vi "Vision_ExecLogic.vi"() -> ()   [LabVIEW 2025]
uses:
  <vilib>/Rock Robotics/WPI/ThirdParty/PhotonVisionLib/Enum/PhotonPoseStrategy_ENUM.ctl
  <vilib>/Rock Robotics/WPI/ThirdParty/JAS_Junk/TrajLib/VI/AprilTagFieldLayout_New2026Welded.vi
  <vilib>/Rock Robotics/WPI/ThirdParty/PhotonVisionLib/SubVI/PhotonPipelineResult_Unpack.vi
  <vilib>/Rock Robotics/WPI/ThirdParty/PhotonVisionLib/SubVI/PhotonPipelineResult_GetMetadata.vi
  <vilib>/Rock Robotics/WPI/ThirdParty/PhotonVisionLib/SubVI/PhotonPipelineMetadata_GetAll.vi
  <vilib>/Rock Robotics/WPI/ThirdParty/PhotonVisionLib/SubVI/PhotonPipelineResult_HasTargets.vi
  <vilib>/Rock Robotics/WPI/ThirdParty/JAS_Junk/TrajLib/VI/Quaternion_New.vi
  <vilib>/Rock Robotics/WPI/ThirdParty/JAS_Junk/TrajLib/VI/AprilTagFieldLayout_New.vi
  <vilib>/Rock Robotics/WPI/ThirdParty/JAS_Junk/TrajLib/VI/Pose3d_New_Trans3dRot3d.vi
  <vilib>/Rock Robotics/WPI/ThirdParty/JAS_Junk/TrajLib/VI/Rotation3d_Create_Quaternion.vi
  <vilib>/Rock Robotics/WPI/ThirdParty/JAS_Junk/TrajLib/VI/AprilTag_New.vi
  <vilib>/Rock Robotics/WPI/ThirdParty/JAS_Junk/TrajLib/VI/Transform3d_Equals.vi
  <vilib>/Rock Robotics/WPI/ThirdParty/PhotonVisionLib/SubVI/PhotonPoseEstimator_SetCamera.vi
  <vilib>/Rock Robotics/WPI/ThirdParty/PhotonVisionLib/SubVI/PhotonPoseEstimator_SetPrimaryStategy.vi
  <vilib>/Rock Robotics/WPI/ThirdParty/PhotonVisionLib/SubVI/PhotonPoseEstimator_SetMultiTagFallbackStrategy.vi
  <vilib>/Rock Robotics/WPI/ThirdParty/PhotonVisionLib/SubVI/PhotonPoseEstimator_SetHighestAmbiguity.vi
  <vilib>/Rock Robotics/WPI/ThirdParty/PhotonVisionLib/SubVI/PhotonPoseEstimator_SetRobotToCameraTransform.vi
  <vilib>/Rock Robotics/WPI/ThirdParty/PhotonVisionLib/SubVI/PhotonPoseEstimator_New.vi
  <vilib>/Rock Robotics/WPI/ThirdParty/PhotonVisionLib/SubVI/PhotonPoseEstimator_SetLastPose.vi
  <vilib>/Rock Robotics/WPI/ThirdParty/PhotonVisionLib/SubVI/PhotonPoseEstimator_SetReferencePose.vi
  <vilib>/Rock Robotics/WPI/ThirdParty/PhotonVisionLib/SubVI/PhotonPoseEstimator_Update_MultiTagOnCoproc.vi
  <vilib>/Rock Robotics/WPI/ThirdParty/PhotonVisionLib/SubVI/PhotonEstimatedRobotPose_GetAll.vi
  <vilib>/Rock Robotics/WPI/ThirdParty/JAS_Junk/TrajLib/VI/Pose3d_ToPose2d.vi
  <vilib>/Rock Robotics/WPI/ThirdParty/PhotonVisionLib/SubVI/Packet_decode_ByteI8.vi
  <vilib>/Rock Robotics/WPI/ThirdParty/PhotonVisionLib/SubVI/PhotonTrackedTarget_Unpack.vi
  <vilib>/Rock Robotics/WPI/ThirdParty/PhotonVisionLib/SubVI/PhotonMultiTargetPNPResult_unpack.vi
  <vilib>/Rock Robotics/WPI/ThirdParty/PhotonVisionLib/SubVI/PhotonPipelineMetadata_Unpack.vi
  <vilib>/Rock Robotics/WPI/ThirdParty/PhotonVisionLib/SubVI/PhotonPipelineResult_New.vi
  <vilib>/Rock Robotics/WPI/ThirdParty/PhotonVisionLib/SubVI/PhotonPipelineResult_GetTargetCount.vi
  <vilib>/Rock Robotics/WPI/ThirdParty/JAS_Junk/TrajLib/VI/AprilTag_GetAll.vi
  <vilib>/Rock Robotics/WPI/ThirdParty/JAS_Junk/TrajLib/VI/Quaternion_Normalize.vi
  <vilib>/Rock Robotics/WPI/ThirdParty/JAS_Junk/TrajLib/VI/Transform3d_GetTranslation3d.vi
  <vilib>/Rock Robotics/WPI/ThirdParty/JAS_Junk/TrajLib/VI/Transform3d_GetRotation3d.vi
  <vilib>/Rock Robotics/WPI/ThirdParty/JAS_Junk/TrajLib/VI/Rotation3d_Equals.vi
  <vilib>/Rock Robotics/WPI/ThirdParty/JAS_Junk/TrajLib/VI/Translation3d_Equals.vi
  <vilib>/Rock Robotics/WPI/ThirdParty/PhotonVisionLib/SubVI/PhotonTargetModel_New_AprilTag36H11.vi
  <vilib>/Rock Robotics/WPI/ThirdParty/JAS_Junk/TrajLib/VI/TimeInterpRotation2d_New.vi
  <vilib>/Rock Robotics/WPI/ThirdParty/PhotonVisionLib/SubVI/PhotonPoseEstimator_GetEmptyPose.vi
  <vilib>/Rock Robotics/WPI/ThirdParty/PhotonVisionLib/SubVI/PhotonPoseEstimator_EstimateMultiTagOnCoprocPose.vi
  <vilib>/Rock Robotics/WPI/ThirdParty/PhotonVisionLib/SubVI/PhotonPipelineResult_GetTimeStampSecs.vi
  <vilib>/Rock Robotics/WPI/ThirdParty/PhotonVisionLib/SubVI/PhotonPoseEstimator_EstimateLowestAmbiguityPose.vi
  <vilib>/Rock Robotics/WPI/ThirdParty/PhotonVisionLib/SubVI/PhotonPoseEstimator_EstimateClosestToCameraHeightPose.vi
  <vilib>/Rock Robotics/WPI/ThirdParty/PhotonVisionLib/SubVI/PhotonPoseEstimator_EstimateClosestToReferencePose.vi
  <vilib>/Rock Robotics/WPI/ThirdParty/PhotonVisionLib/SubVI/PhotonPoseEstimator_GetReferencePose.vi
  <vilib>/Rock Robotics/WPI/ThirdParty/PhotonVisionLib/SubVI/PhotonPoseEstimator_GetLastPose.vi
  <vilib>/Rock Robotics/WPI/ThirdParty/PhotonVisionLib/SubVI/PhotonPoseEstimator_EstimateAverageBestTargetsPose.vi
  <vilib>/Rock Robotics/WPI/ThirdParty/PhotonVisionLib/SubVI/PhotonEstimatedRobotPose_New.vi
  <vilib>/Rock Robotics/WPI/ThirdParty/PhotonVisionLib/SubVI/PhotonPoseEstimator_EstimatePnpDistanceTrigSolvePose.vi
  <vilib>/Rock Robotics/WPI/ThirdParty/PhotonVisionLib/SubVI/PhotonPoseEstimator_ShouldEstimate.vi
  <vilib>/Rock Robotics/WPI/ThirdParty/JAS_Junk/TrajLib/VI/Pose3d_getTranslation3d.vi
  <vilib>/Rock Robotics/WPI/ThirdParty/JAS_Junk/TrajLib/VI/Pose3d_getRotation3d.vi
  <vilib>/Rock Robotics/WPI/ThirdParty/JAS_Junk/TrajLib/VI/Translation3d_ToTranslation2d.vi
  <vilib>/Rock Robotics/WPI/ThirdParty/JAS_Junk/TrajLib/VI/Rotation3d_ToRotation2d.vi
  <vilib>/Rock Robotics/WPI/ThirdParty/JAS_Junk/TrajLib/Pose2d_New_TRRO.vi
  <vilib>/Rock Robotics/WPI/ThirdParty/PhotonVisionLib/SubVI/Packet_decode_Flt64.vi
  <vilib>/Rock Robotics/WPI/ThirdParty/PhotonVisionLib/SubVI/TargetCorner_New.vi
  <vilib>/Rock Robotics/WPI/ThirdParty/PhotonVisionLib/SubVI/Packet_decode_Int32.vi
  <vilib>/Rock Robotics/WPI/ThirdParty/PhotonVisionLib/SubVI/Packet_decode_Transform3d.vi
  <vilib>/Rock Robotics/WPI/ThirdParty/PhotonVisionLib/SubVI/Packet_decode_Flt32.vi
  <vilib>/Rock Robotics/WPI/ThirdParty/PhotonVisionLib/SubVI/Packet_decode_TargetCornerArray.vi
  <vilib>/Rock Robotics/WPI/ThirdParty/PhotonVisionLib/SubVI/Packet_decode_Boolean.vi
  <vilib>/Rock Robotics/WPI/ThirdParty/PhotonVisionLib/SubVI/PhotonPNPResult_unpack.vi
  <vilib>/Rock Robotics/WPI/ThirdParty/PhotonVisionLib/SubVI/PhotonMultiTargetPNPResult_New.vi
  <vilib>/Rock Robotics/WPI/ThirdParty/PhotonVisionLib/SubVI/Packet_decode_Int16.vi
  <vilib>/Rock Robotics/WPI/ThirdParty/PhotonVisionLib/SubVI/Packet_decode_Int64.vi
  <vilib>/Rock Robotics/WPI/ThirdParty/JAS_Junk/TrajLib/VI/Quaternion_New_Default.vi
  <vilib>/Rock Robotics/WPI/ThirdParty/JAS_Junk/TrajLib/VI/Rotation3d_GetQuaterion.vi
  <vilib>/Rock Robotics/WPI/ThirdParty/JAS_Junk/TrajLib/VI/Quaternion_Equals.vi
  <vilib>/Rock Robotics/WPI/ThirdParty/PhotonVisionLib/SubVI/PhotonTargetModel_New_RectPlanar.vi
  <vilib>/Rock Robotics/WPI/ThirdParty/JAS_Junk/TrajLib/Conv_Inches_Meters.vi
  <vilib>/Rock Robotics/WPI/ThirdParty/JAS_Junk/TrajLib/VI/Rotation3d_Create_AxisAngle.vi
  <vilib>/Rock Robotics/WPI/ThirdParty/JAS_Junk/TrajLib/VI/Pose3d_New.vi
  <vilib>/Rock Robotics/WPI/ThirdParty/JAS_Junk/TrajLib/VI/Pose3d_New_Default.vi
  <vilib>/Rock Robotics/WPI/ThirdParty/JAS_Junk/TrajLib/VI/Pose3d_Plus.vi
  <vilib>/Rock Robotics/WPI/ThirdParty/JAS_Junk/TrajLib/VI/Pose3d_RelativeTo.vi
  <vilib>/Rock Robotics/WPI/ThirdParty/PhotonVisionLib/SubVI/PhotonPoseEstimator_GetFieldTags.vi
  <vilib>/Rock Robotics/WPI/ThirdParty/JAS_Junk/TrajLib/VI/AprilTagFieldLayout_GetOriginPosition.vi
  <vilib>/Rock Robotics/WPI/ThirdParty/JAS_Junk/TrajLib/VI/Transform3d_Inverse.vi
  <vilib>/Rock Robotics/WPI/ThirdParty/PhotonVisionLib/SubVI/PhotonPoseEstimator_GetRobotToCameraTransform.vi
  <vilib>/Rock Robotics/WPI/ThirdParty/PhotonVisionLib/SubVI/PhotonPipelineResult_GetTargets.vi
  <vilib>/Rock Robotics/WPI/ThirdParty/PhotonVisionLib/SubVI/PhotonPipelineResult_GetMultiTagResult.vi
  <vilib>/Rock Robotics/WPI/ThirdParty/PhotonVisionLib/SubVI/PhotonTrackedTarget_GetPoseAmbiguity.vi
  <vilib>/Rock Robotics/WPI/ThirdParty/PhotonVisionLib/SubVI/PhotonTrackedTarget_GetFiducialId.vi
  <vilib>/Rock Robotics/WPI/ThirdParty/JAS_Junk/TrajLib/VI/AprilTagFieldLayout_GetTagPose.vi
  <vilib>/Rock Robotics/WPI/ThirdParty/JAS_Junk/TrajLib/VI/Pose3d_TransformBy.vi
  <vilib>/Rock Robotics/WPI/ThirdParty/PhotonVisionLib/SubVI/PhotonTrackedTarget_GetBestCameraToTarget.vi
  <vilib>/Rock Robotics/WPI/ThirdParty/PhotonVisionLib/SubVI/PhotonPoseEstimator_GetHighestAmbiguity.vi
  <vilib>/Rock Robotics/WPI/ThirdParty/PhotonVisionLib/SubVI/PhotonPoseEstimator_Strategy_closestToCameraHeight_calc.vi
  <vilib>/Rock Robotics/WPI/ThirdParty/PhotonVisionLib/SubVI/PhotonTrackedTarget_GetAltCameraToTarget.vi
  <vilib>/Rock Robotics/WPI/ThirdParty/PhotonVisionLib/SubVI/PhotonPoseEstimator_Strategy_closestToReferencePose_calc.vi
  <vilib>/Rock Robotics/WPI/ThirdParty/PhotonVisionLib/SubVI/PhotonPoseEstimator_Strategy_averageBestTargets_calc.vi
  <vilib>/Rock Robotics/WPI/ThirdParty/JAS_Junk/TrajLib/VI/Rotation3d_Plus.vi
  <vilib>/Rock Robotics/WPI/ThirdParty/JAS_Junk/TrajLib/VI/Translation3d_Plus.vi
  <vilib>/Rock Robotics/WPI/ThirdParty/JAS_Junk/TrajLib/VI/Translation3d_Times.vi
  <vilib>/Rock Robotics/WPI/ThirdParty/JAS_Junk/TrajLib/VI/Rotation3d_Times.vi
  <vilib>/Rock Robotics/WPI/ThirdParty/JAS_Junk/TrajLib/VI/Rotation3d_Create_Default.vi
  <vilib>/Rock Robotics/WPI/ThirdParty/JAS_Junk/TrajLib/VI/Translation3d_Create_Default.vi
  <vilib>/Rock Robotics/WPI/ThirdParty/JAS_Junk/TrajLib/VI/Translation3d_GetNorm.vi
  <vilib>/Rock Robotics/WPI/ThirdParty/JAS_Junk/TrajLib/VI/Translation3d_Create_DistAng.vi
  <vilib>/Rock Robotics/WPI/ThirdParty/JAS_Junk/TrajLib/VI/Translation3d_RotateBy.vi
  <vilib>/Rock Robotics/WPI/ThirdParty/JAS_Junk/TrajLib/Translation2d_RotateBy.vi
  <vilib>/Rock Robotics/WPI/ThirdParty/JAS_Junk/TrajLib/Pose2d_getTranslation.vi
  <vilib>/Rock Robotics/WPI/ThirdParty/JAS_Junk/TrajLib/Translation2d_Plus.vi
  <vilib>/Rock Robotics/WPI/ThirdParty/JAS_Junk/TrajLib/Translation2d_UnaryMinus.vi
  <vilib>/Rock Robotics/WPI/ThirdParty/JAS_Junk/TrajLib/VI/Pose3d_New_Pose2d.vi
  <vilib>/Rock Robotics/WPI/ThirdParty/JAS_Junk/TrajLib/VI/TimeInterpRotation2d_GetSample.vi
  <vilib>/Rock Robotics/WPI/ThirdParty/PhotonVisionLib/SubVI/PhotonPoseEstimator_GetHeadingBuffer.vi
  <vilib>/Rock Robotics/WPI/ThirdParty/JAS_Junk/TrajLib/Translation2d_Create.vi
  <vilib>/Rock Robotics/WPI/ThirdParty/JAS_Junk/TrajLib/Rotation2d_CreateAngle.vi
  <vilib>/Rock Robotics/WPI/ThirdParty/JAS_Junk/TrajLib/VI/Rotation3d_GetXYZ.vi
  <vilib>/Rock Robotics/WPI/ThirdParty/PhotonVisionLib/SubVI/PhotonPNPResult_New.vi
  <vilib>/Rock Robotics/WPI/ThirdParty/JAS_Junk/TrajLib/VI/Quaternion_Get_Vect.vi
  <vilib>/Rock Robotics/WPI/ThirdParty/JAS_Junk/TrajLib/VI/Quaternion_Get_W.vi
  <vilib>/Rock Robotics/WPI/ThirdParty/PhotonVisionLib/SubVI/PhotonTargetModel_New.vi
  <vilib>/Rock Robotics/WPI/ThirdParty/JAS_Junk/TrajLib/VI/Vector_Norm.vi
  <vilib>/Rock Robotics/WPI/ThirdParty/JAS_Junk/TrajLib/VecBuilder_ArrayBy1Fill.vi
  <vilib>/Rock Robotics/WPI/ThirdParty/JAS_Junk/TrajLib/VI/Transform3d_Create_Pose3dPose3d.vi
  <vilib>/Rock Robotics/WPI/ThirdParty/JAS_Junk/TrajLib/VI/Rotation3d_UnaryMinus.vi
  <vilib>/Rock Robotics/WPI/ThirdParty/JAS_Junk/TrajLib/VI/Translation3d_UnaryMinus.vi
  <vilib>/Rock Robotics/WPI/ThirdParty/JAS_Junk/TrajLib/Transform2d_Create_TransRot.vi
  <vilib>/Rock Robotics/WPI/ThirdParty/JAS_Junk/TrajLib/VI/Transform3d_GetXYZ.vi
  <vilib>/Rock Robotics/WPI/ThirdParty/JAS_Junk/TrajLib/VI/Pose3d_getXYZ.vi
  <vilib>/Rock Robotics/WPI/ThirdParty/PhotonVisionLib/SubVI/PhotonPoseEstimator_CalcDifference.vi
  <vilib>/Rock Robotics/WPI/ThirdParty/JAS_Junk/TrajLib/VI/Rotation3d_RotateBy.vi
  <vilib>/Rock Robotics/WPI/ThirdParty/JAS_Junk/TrajLib/VI/Translation3d_GetXYZ.vi
  <vilib>/Rock Robotics/WPI/ThirdParty/JAS_Junk/TrajLib/VI/Quaternion_Times.vi
  <vilib>/Rock Robotics/WPI/ThirdParty/JAS_Junk/TrajLib/VI/Quaternion_Inverse.vi
  <vilib>/Rock Robotics/WPI/ThirdParty/JAS_Junk/TrajLib/VI/Quaternion_Get_All.vi
  <vilib>/Rock Robotics/WPI/ThirdParty/JAS_Junk/TrajLib/Rotation2d_Interpolate.vi
  <vilib>/Rock Robotics/WPI/ThirdParty/JAS_Junk/TrajLib/MatBuilder_Create.vi
  <vilib>/Rock Robotics/WPI/ThirdParty/JAS_Junk/TrajLib/VI/Translation3d_Minus.vi
  <vilib>/Rock Robotics/WPI/ThirdParty/JAS_Junk/TrajLib/VI/Rotation3d_Minus.vi
  <vilib>/Rock Robotics/WPI/ThirdParty/JAS_Junk/TrajLib/VI/Translation3d_GetDistance.vi
  <vilib>/Rock Robotics/WPI/ThirdParty/JAS_Junk/TrajLib/Rotation2d_Plus.vi
  <vilib>/Rock Robotics/WPI/ThirdParty/JAS_Junk/TrajLib/Rotation2d_Minus.vi
  <vilib>/Rock Robotics/WPI/ThirdParty/JAS_Junk/TrajLib/MathUtil_Clamp.vi
  <vilib>/Rock Robotics/WPI/ThirdParty/JAS_Junk/TrajLib/Rotation2d_Times.vi
  <vilib>/Rock Robotics/WPI/ThirdParty/JAS_Junk/TrajLib/Rotation2d_RotateBy.vi
  <vilib>/Rock Robotics/WPI/ThirdParty/JAS_Junk/TrajLib/Rotation2d_UnaryMinus.vi
  <vilib>/Rock Robotics/WPI/ThirdParty/JAS_Junk/TrajLib/Rotation2d_CreateXY.vi
  <vilib>/Rock Robotics/WPI/ThirdParty/JAS_Junk/TrajLib/Util_CalcDist.vi
  <vilib>/Rock Robotics/Network Tables/NT Read Value.vi
  <vilib>/Rock Robotics/Network Tables/NT Read Raw.vi
  <vilib>/Rock Robotics/WPI/ThirdParty/PhotonVisionLib/SubVI/PhotonVision_Globals.vi
  <vilib>/gmath/interp.llb/Search Ordered Table.vi
  <vilib>/Rock Robotics/Network Tables/NT Write Number.vi
  <vilib>/Rock Robotics/Network Tables/NT Write Boolean.vi
  <vilib>/Rock Robotics/WPI/ThirdParty/PhotonVisionLib/PhotonVisionLib.lvlib
  <vilib>/Rock Robotics/WPI/ThirdParty/JAS_Junk/TrajLib/Trajectory_Library.lvlib
panel:
  in  "Drive Encoder  Dstance (Meters)":dbl
  in  "Gyro Reading (Deg)":dbl
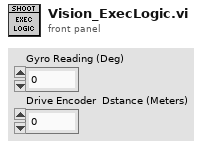
[diagram p1: front panel]
types:
  T1 = typedef "PhotonVisionLib.lvlib/PhotonPoseStrategy_ENUM.ctl" = enum16{"LOWEST_AMBIGUITY", "CLOSEST_TO_CAMERA_HEIGHT", "CLOSEST_TO_REFERENCE_POSE", "CLOSEST_TO_LAST_POSE", "AVERAGE_BEST_TARGETS", "MULTI_TAG_PNP_ON_COPROCESSOR", "MULTI_TAG_PNP_ON_RIO", "PNP_DISTANCE_TRIG_SOLVE", "CONSTRAINED_SOLVEPNP"}
  T2 = typedef "Trajectory_Library.lvlib/TRANSLATION3D.ctl" = cluster{"X":dbl, "Y":dbl, "Z":dbl}
  T3 = typedef "Trajectory_Library.lvlib/AprilTagFieldLayout.ctl" = cluster{"AprilTagMap":map{i32, T4}, "FieldLength":dbl, "FieldWidth":dbl, "OriginPosition ":T8, "OriginPose3d":T5}
  T4 = typedef "Trajectory_Library.lvlib/AprilTag.ctl" = cluster{"ID":i32, "POSE3D":T5}
  T5 = typedef "Trajectory_Library.lvlib/POSE3D.ctl" = cluster{"Translation3d":T2, "Rotation3d":T6}
  T6 = typedef "Trajectory_Library.lvlib/ROTATION3D.ctl" = cluster{"Q_quaternion":T7}
  T7 = typedef "Trajectory_Library.lvlib/QUATERNION.ctl" = cluster{"R":dbl, "V":dbl[]}
  T8 = typedef "Trajectory_Library.lvlib/AprilTagFieldLayoutOrignPosition_ENUM.ctl" = enum16{"kBlueAllianceWallRightSide,", "kRedAllianceWallRightSide,"}
  T9 = typedef "PhotonVisionLib.lvlib/PhotonPipelineResultType.ctl" = cluster{"Targets":T10[], "PhotonMultiTargetPNPResult":T13, "PhotonPipelineMetadata":T15}
  T10 = typedef "PhotonVisionLib.lvlib/PhotonTrackedTargetType.ctl" = cluster{"Yaw":dbl, "Pitch":dbl, "Area":dbl, "Skew":dbl, "MinAreaRectCorners":T11[], "BestCameraToTarget":T12, "FiducialId":i32, "AltCameraToTarget":T12, "PoseAmbiguity":dbl, "DetectedCorners":T11[], "ObjDetectId":i32, "ObjDetectConf":sgl}
  T11 = typedef "PhotonVisionLib.lvlib/TargetCornerType.ctl" = cluster{"X":dbl, "Y":dbl}
  T12 = typedef "Trajectory_Library.lvlib/TRANSFORM3D.ctl" = cluster{"TRANSLATION3D":T2, "ROTATION3D":T6, "XF":bool}
  T13 = typedef "PhotonVisionLib.lvlib/PhotonMultiTargetPNPResultType.ctl" = cluster{"PhotonPNPResult":T14, "FiducialIDsUsed":i16[]}
  T14 = typedef "PhotonVisionLib.lvlib/PhotonPNPResultType.ctl" = cluster{"IsPresent":bool, "bestReprojErr":dbl, "altReprojErr":dbl, "ambiguity":dbl, "Best":T12, "Alt":T12}
  T15 = typedef "PhotonVisionLib.lvlib/PhotonPipelineMetadataType.ctl" = cluster{"CaptureTimestampMicros":i64, "PublishTimestampMicros":i64, "SequenceID":i64, "TimeSinceLastPong":i64}
  T16 = typedef "PhotonVisionLib.lvlib/PhotonPoseEstimator_Configuration.ctl" = cluster{"Primary Strategy":T1, "Camera":string, "Initial Pose":T5, "HighestAmbiguity":dbl, "RobotToCamera":T12, "FallBack Strategy":T1, "BaseNTName":string}
  T17 = typedef "Trajectory_Library.lvlib/POSE2D.ctl" = cluster{"TRANSLATION":T18, "ROTATION":T19}
  T18 = typedef "Trajectory_Library.lvlib/TRANSLATION2D.ctl" = cluster{"X":dbl, "Y":dbl}
  T19 = typedef "Trajectory_Library.lvlib/ROTATION2D.ctl" = cluster{"VALUE":dbl, "COS":dbl, "SIN":dbl}
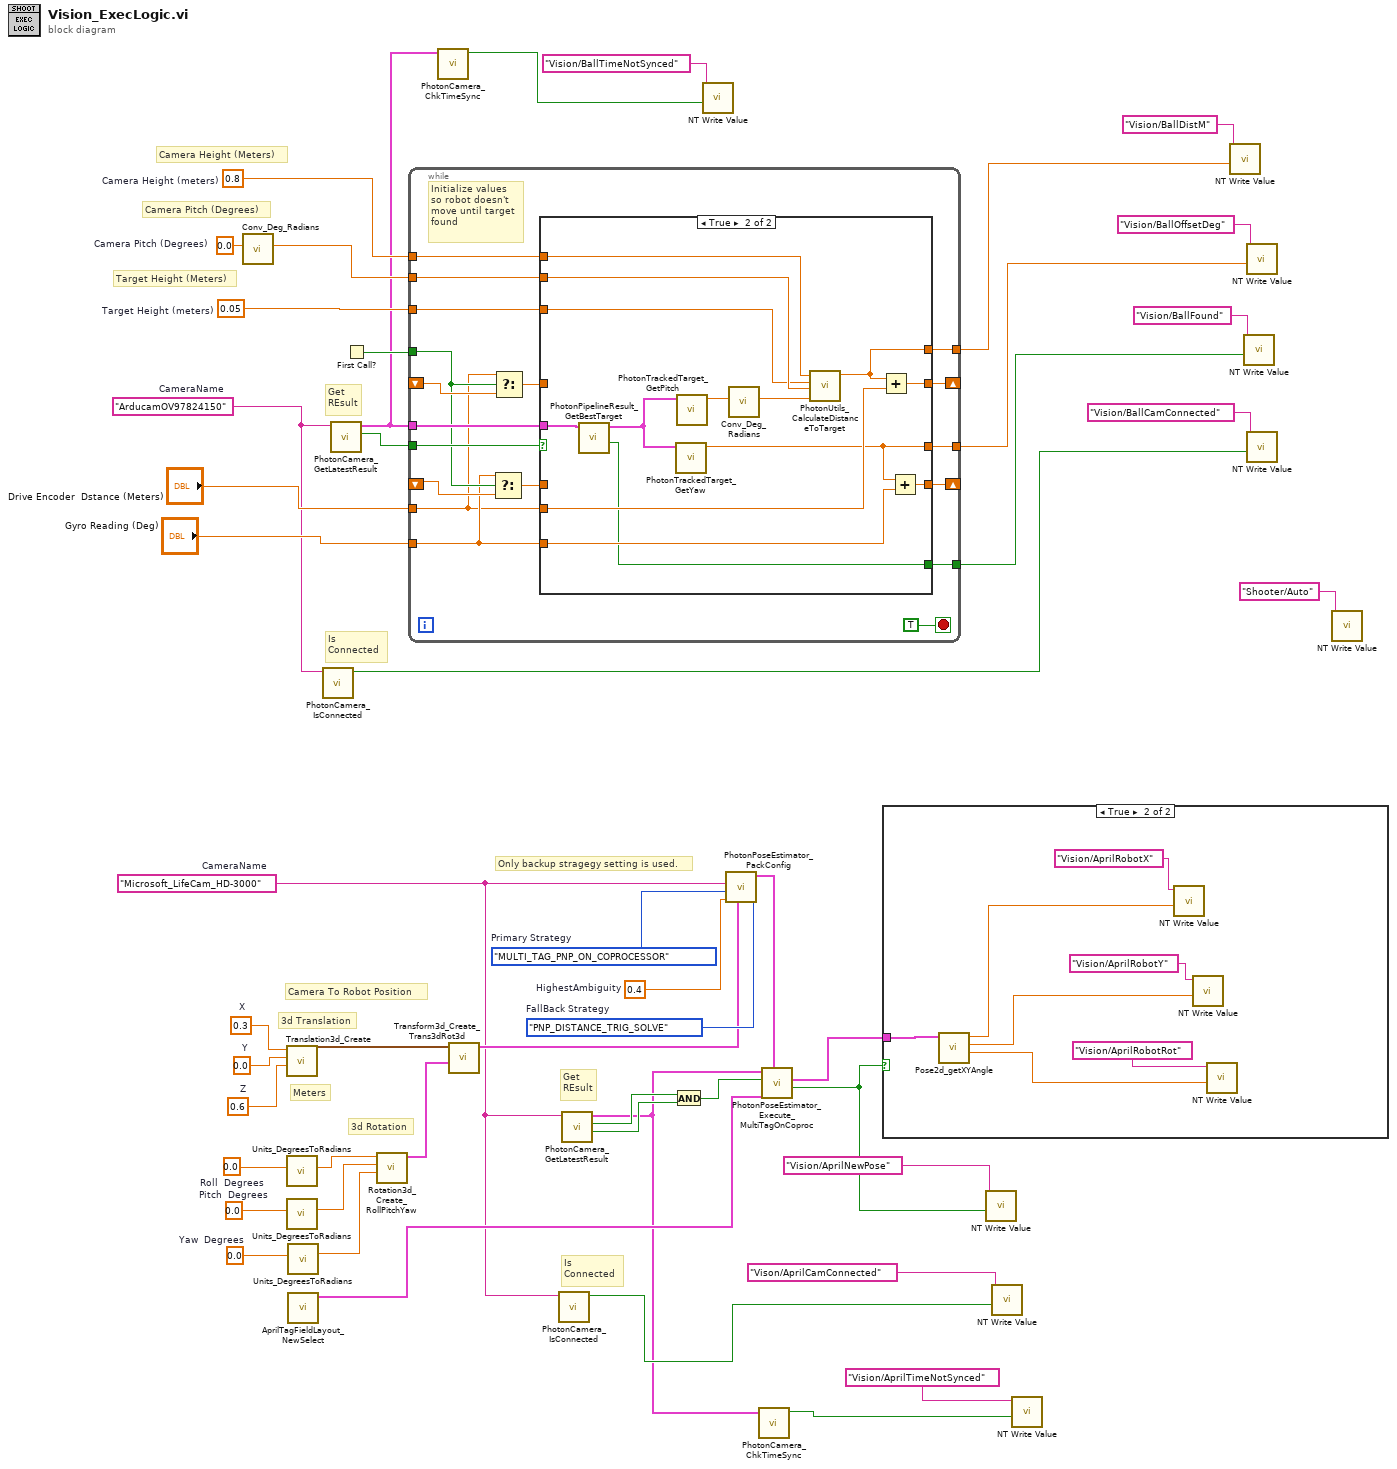
[diagram p0: block diagram]
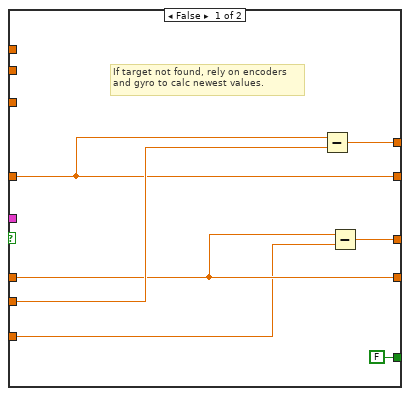
[diagram p3: hidden frame]
diagram:
  w29 = PhotonPoseStrategy_ENUM."PNP_DISTANCE_TRIG_SOLVE"  # FallBack Strategy
  w22 = 0.0  # Roll  Degrees
  w21 = 0.0  # Pitch  Degrees
  w20 = 0.0  # Yaw  Degrees
  w14 = 0.6  # Z
  w15 = 0.3  # X
  w16 = 0.0  # Y
  w13 = 0.4  # HighestAmbiguity
  w12 = PhotonPoseStrategy_ENUM."MULTI_TAG_PNP_ON_COPROCESSOR"  # Primary Strategy
  w11 = "Microsoft_LifeCam_HD-3000"  # CameraName
  w42 = 0.05  # Target Height (meters)
  w40 = 0.8  # Camera Height (meters)
  w38 = 0.0  # Camera Pitch (Degrees)
  w37 = "ArducamOV97824150"  # CameraName
  # "Only backup stragegy setting is used."
  # "Meters"
  # "Camera To Robot Position"
  # "3d Rotation"
  # "3d Translation"
  # "Is\nConnected"
  # "Get\nREsult"
  # "Camera Pitch (Degrees)"
  # "Target Height (Meters)"
  # "Camera Height (Meters)"
  # "Is\nConnected"
  # "Get\nREsult"
  n1 = call <vilib>:"Conv_Deg_Radians.vi"("Degress"=w38) -> ("Radians"=w41:dbl)  [unwired: 10 in]
  n2 = call <vilib>:"Translation3d_Create.vi"("Z"=w14, "Y"=w16, "X"=w15) -> ("TRANSLATION3D"=w23:T2)  [unwired: 8 in]
  n3 = call <vilib>:"Units_DegreesToRadians.vi"("Degrees"=w22) -> ("Radians"=w19:dbl)  [unwired: 10 in]
  n4 = call <vilib>:"Units_DegreesToRadians.vi"("Degrees"=w21) -> ("Radians"=w18:dbl)  [unwired: 10 in]
  n5 = call <vilib>:"Units_DegreesToRadians.vi"("Degrees"=w20) -> ("Radians"=w17:dbl)  [unwired: 10 in]
  n6 = call-poly <vilib>:"AprilTagFieldLayout_NewSelect.vi"() -> ("AprilTagFieldLayout"=w30:T3)  [unwired: 11 in]
  n7 = call <vilib>:"PhotonCamera_IsConnected.vi"("CameraName"=w37) -> ("IsConnected"=w31:bool)  [unwired: 9 in, 1 out]
  n8 = call <vilib>:"PhotonCamera_GetLatestResult.vi"("CameraName"=w37) -> ("HasTargets"=w39:bool, "PipelineResult"=w6:T9)  [unwired: 6 in, 3 out]
  n9 = First Call?() -> (First Call?: T/F=w45:bool)
  n10 = call <vilib>:"Rotation3d_Create_RollPitchYaw.vi"("Yaw"=w17, "Pitch"=w18, "Roll"=w19) -> ("Rotation3d"=w24:T6)  [unwired: 8 in]
  n11 = while {
    tunnel: w39 -> [w68]
    tunnel: w6 -> [w67]
    tunnel: w40 -> [w66]
    tunnel: w41 -> [w65]
    tunnel: w42 -> [w64]
    tunnel: [w63] -> w36
    tunnel: [w62] -> w35
    tunnel: "Drive Encoder  Dstance (Meters)" -> [w51]
    shift-right: [w60] -> _
    shift-left: _ -> [w58]
    tunnel: "Gyro Reading (Deg)" -> [w52]
    shift-right: [w59] -> _
    shift-left: _ -> [w56]
    tunnel: w45 -> [w54]
    tunnel: [w53] -> w33
    stop <- TRUE stop-if-true
    # "Initialize values\nso robot doesn't\nmove until target\nfound"
    n12 = Select(t=w52, s=w54, f=w56) -> (s? t:f=w55:dbl)
    n13 = Select(t=w51, s=w54, f=w58) -> (s? t:f=w57:dbl)
    n14 = case shown="True" w68 {
      tunnel: w67 -> [_ w89]
      tunnel: [w72 w79] -> w62
      tunnel: w66 -> [_ w85]
      tunnel: w65 -> [_ w84]
      tunnel: w64 -> [_ w83]
      tunnel: [w74 w82] -> w63
      tunnel: w51 -> [w75 w81]
      tunnel: [w73 w80] -> w60
      tunnel: w57 -> [w73 _]
      tunnel: w52 -> [w70 w78]
      tunnel: [w71 w77] -> w59
      tunnel: w55 -> [w71 _]
      tunnel: [FALSE ("TargetFound") w76] -> w53
      frame False {
        # "If target not found, rely on encoders\nand gyro to calc newest values."
        n15 = Subtract(x=w73, y=w75) -> (x-y=w74:dbl)
        n16 = Subtract(x=w71, y=w70) -> (x-y=w72:dbl)
      }
      frame True {
        n17 = call <vilib>:"PhotonPipelineResult_GetBestTarget.vi"("PhotonPipelineResult"=w89) -> ("TargetFound"=w76:bool, "PhotonTrackedTarget"=w88:T10)  [unwired: 9 in]
        n18 = call <vilib>:"PhotonTrackedTarget_GetYaw.vi"("TrackedTarget"=w88) -> ("Yaw"=w79:dbl)  [unwired: 10 in]
        n19 = call <vilib>:"PhotonTrackedTarget_GetPitch.vi"("TrackedTarget"=w88) -> ("Pitch"=w87:dbl)  [unwired: 10 in]
        n20 = call <vilib>:"Conv_Deg_Radians.vi"("Degress"=w87) -> ("Radians"=w86:dbl)  [unwired: 10 in]
        n21 = call <vilib>:"PhotonUtils_CalculateDistanceToTarget.vi"("TargetPitch_Radians"=w86, "CameraPitch_Radians"=w84, "TargetHeight_Meters"=w83, "CameraHeight_Meters"=w85) -> ("DistanceToTarget_Meters"=w82:dbl)  [unwired: 7 in]
        n22 = Add(x=w82, y=w81) -> (x+y=w80:dbl)
        n23 = Add(x=w79, y=w78) -> (x+y=w77:dbl)
      }
    }
  }
  n24 = call <vilib>:"PhotonCamera_ChkTimeSync.vi"("PhotonPipelineResult"=w6) -> ("TimeNotSynced"=w4:bool)  [unwired: 10 in]
  n25 = call <vilib>:"Transform3d_Create_Trans3dRot3d.vi"("Rotation3d"=w24, "Translation3d"=w23) -> ("Transform3d"=w25:T12)  [unwired: 9 in]
  n26 = call <vilib>:"PhotonCamera_IsConnected.vi"("CameraName"=w11) -> ("IsConnected"=w9:bool)  [unwired: 9 in, 1 out]
  n27 = call <vilib>:"PhotonCamera_GetLatestResult.vi"("CameraName"=w11) -> ("New Data"=w28:bool, "HasTargets"=w27:bool, "PipelineResult"=w1:T9)  [unwired: 6 in, 2 out]
  n28 = And(x=w27, y=w28) -> (x .and. y?=w26:bool)
  n29 = call-poly <vilib>:"NT Write Value.vi"("value"=w4, "name"="Vision/BallTimeNotSynced") -> ()  [unwired: 9 in, 1 out]
  n30 = call <vilib>:"PhotonPoseEstimator_PackConfig.vi"("FallBack Strategy"=w29, "RobotToCamera"=w25, "HighestAmbiguity"=w13, "PirmaryStrategy"=w12, "Camera"=w11) -> ("PoseEstimator_Configuration"=w10:T16)  [unwired: 6 in]
  n31 = call <vilib>:"PhotonCamera_ChkTimeSync.vi"("PhotonPipelineResult"=w1) -> ("TimeNotSynced"=w2:bool)  [unwired: 10 in]
  n32 = call <vilib>:"PhotonPoseEstimator_Execute_MultiTagOnCoproc.vi"("Configuration"=w10, "AprilTagFieldLayout"=w30, "PIpeline Has \nNew Results"=w26, "PipelineResult"=w1) -> ("New Pose Found"=w7:bool, "EstimatedPose2d"=w8:T17)  [unwired: 1 in, 5 out]
  n33 = case shown="True" w7 {
    tunnel: w8 -> [_ w96]
    frame False {
    }
    frame True {
      n34 = call <vilib>:"Pose2d_getXYAngle.vi"("in POSE"=w96) -> ("Angle"=w90:dbl, "Y"=w91:dbl, "X"=w92:dbl)  [unwired: 8 in]
      n35 = call-poly <vilib>:"NT Write Value.vi"("value"=w92, "name"="Vision/AprilRobotX") -> ()  [unwired: 9 in, 1 out]
      n36 = call-poly <vilib>:"NT Write Value.vi"("value"=w91, "name"="Vision/AprilRobotY") -> ()  [unwired: 9 in, 1 out]
      n37 = call-poly <vilib>:"NT Write Value.vi"("value"=w90, "name"="Vision/AprilRobotRot") -> ()  [unwired: 9 in, 1 out]
    }
  }
  n38 = call-poly <vilib>:"NT Write Value.vi"("value"=w7, "name"="Vision/AprilNewPose") -> ()  [unwired: 9 in, 1 out]
  n39 = call-poly <vilib>:"NT Write Value.vi"("value"=w9, "name"="Vison/AprilCamConnected") -> ()  [unwired: 9 in, 1 out]
  n40 = call-poly <vilib>:"NT Write Value.vi"("value"=w2, "name"="Vision/AprilTimeNotSynced") -> ()  [unwired: 9 in, 1 out]
  n41 = call-poly <vilib>:"NT Write Value.vi"("value"=w36, "name"="Vision/BallDistM") -> ()  [unwired: 9 in, 1 out]
  n42 = call-poly <vilib>:"NT Write Value.vi"("value"=w33, "name"="Vision/BallFound") -> ()  [unwired: 9 in, 1 out]
  n43 = call-poly <vilib>:"NT Write Value.vi"("value"=w35, "name"="Vision/BallOffsetDeg") -> ()  [unwired: 9 in, 1 out]
  n44 = call-poly <vilib>:"NT Write Value.vi"("value"=w31, "name"="Vision/BallCamConnected") -> ()  [unwired: 9 in, 1 out]
  n45 = call-poly <vilib>:"NT Write Value.vi"("name"="Shooter/Auto") -> ()  [unwired: 10 in, 1 out]
